vi "Frame Get bp.vi"(8 "error in (no error)":errorcluster, 11 "IDE simple in":refnum<class "Main Panel.lvclass">) -> (0 "error out":errorcluster, 2 "<bp> Data":T1, 3 "IDE simple out":refnum<class "Main Panel.lvclass">)   [LabVIEW 2018, in "Main Panel.lvlib" / "Main Panel.lvclass"]
uses:
  Main Panel.lvclass
  Frame Analizer/frame bp data.ctl
  Main Panel.lvclass/Main Panel.ctl
  Frame Analizer/Data Parser.lvclass
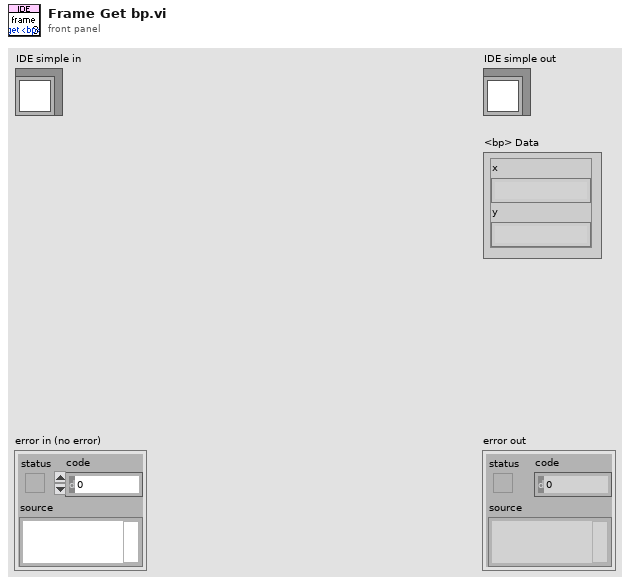
[diagram p1: front panel]
types:
  T1 = typedef "Data Parser.lvclass/frame bp data.ctl" = cluster{"x":string, "y":string}
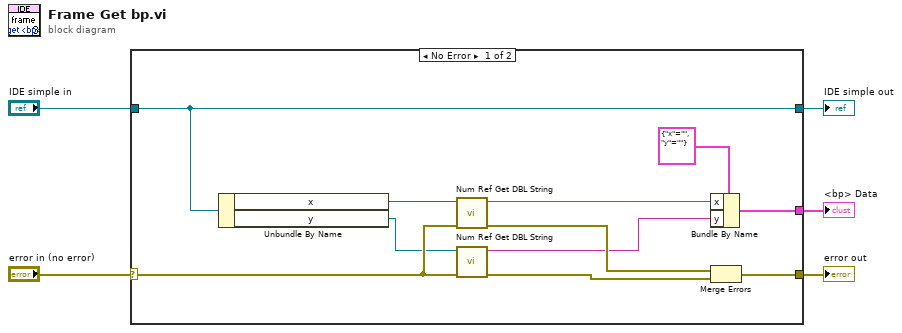
[diagram p0: block diagram]
diagram:
  n1 = case shown="No Error" "error in (no error)" {
    selector: "error in (no error)" -> [w12 w18]
    tunnel: [w16 w18] -> w4
    tunnel: [w8 w17] -> w2
    tunnel: "IDE simple in" -> [w8 w17]
    tunnel: [w15 _] -> w1
    frame No Error {
      n2 = Unbundle By Name(w8) -> ("x"=w7:refnum<vi>, "y"=w6:refnum<vi>)
      n3 = call "Num Ref Get DBL String.vi"("error in (no error)"=w12, "DBL Ref"=w7) -> ("error out"=w11:errorcluster, "Value string"=w13:string)  [unwired: 8 in]
      n4 = call "Num Ref Get DBL String.vi"("error in (no error)"=w12, "DBL Ref"=w6) -> ("error out"=w10:errorcluster, "Value string"=w9:string)  [unwired: 8 in]
      n5 = Bundle By Name(cluster=T1 {"x"="", "y"=""} ("<bp> data 2"), "x"=w13, "y"=w9) -> (w15:T1)
      n6 = Merge Errors(w11, w10) -> (w16:errorcluster)
    }
    frame Error {
    }
  }
  "error out" <- w4
  "IDE simple out" <- w2
  "<bp> Data" <- w1
